vi "Flush Group Buffer.vi"(0 "TDMS File Ref in":refnum<k34>, 5 "Group Name":string, 7 "Channels":string[](array[string]), 9 "Group Buffer Data in":T1, 11 "error in (no error)":errorcluster) -> (4 "TDMS File Ref out":refnum<k34>, 8 "Flushed Data Size":u32, 10 "Group Buffer Data out":T1, 15 "error out":errorcluster)   [LabVIEW 2027, in "Embedded Data Logger Engine.lvlib"]
uses:
  Embedded Data Logger Engine.lvlib
  Group Buffer Data.ctl
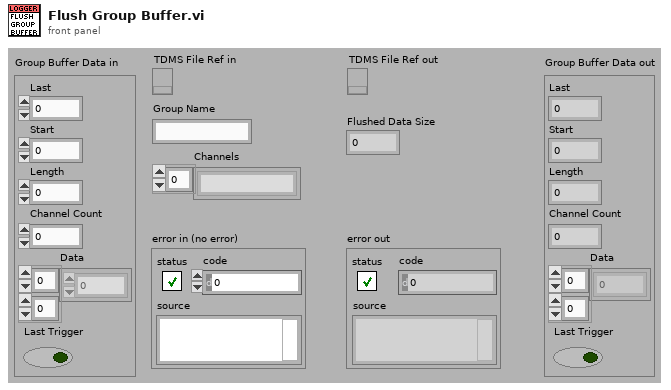
[diagram p1: front panel]
types:
  T1 = typedef "Embedded Data Logger Engine.lvlib/Group Buffer Data.ctl" = cluster{"Last":i32, "Start":i32, "Length":i32, "Channel Count":i32, "Data":dbl[][], "Last Trigger":bool}
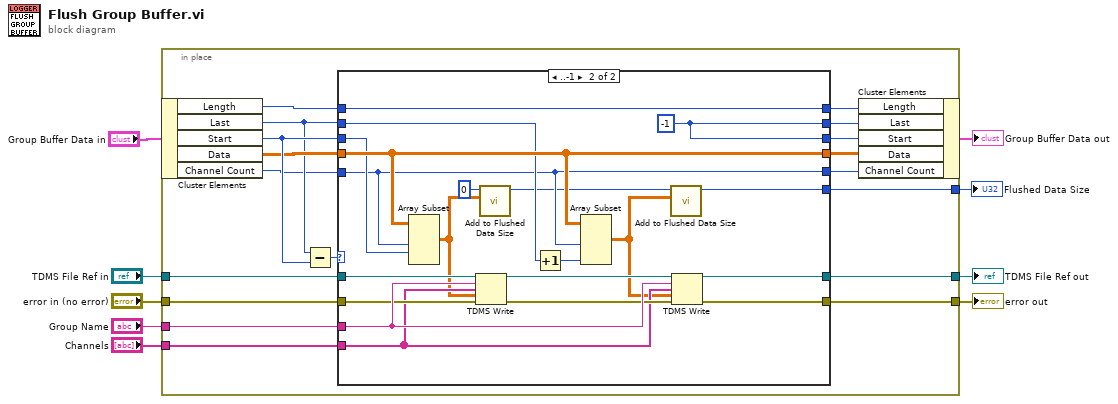
[diagram p0: block diagram]
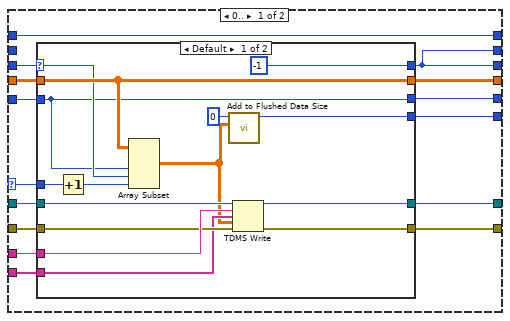
[diagram p2: hidden frame]
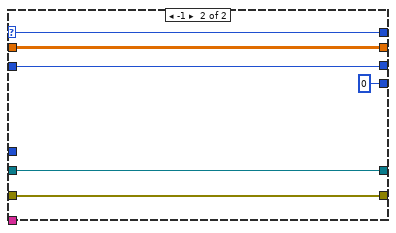
[diagram p3: hidden frame]
diagram:
  n1 = in-place {
    in-place-border: "error in (no error)" -> [w23]
    in-place-border: "TDMS File Ref in" -> [w26]
    in-place-border: [w25] -> w5
    in-place-border: [w24] -> w4
    in-place-border: "Group Name" -> [w22]
    in-place-border: "Channels" -> [w21]
    in-place-border: [w10] -> w1
    n2 = in-place-cluster #1("Group Buffer Data in") -> ("Length"=w14:i32, "Last"=w17:i32, "Start"=w27:i32, "Data"=w20:dbl[][], "Channel Count"=w11:i32)
    n3 = Subtract(x=w17, y=w27) -> (x-y=w18:i32)
    n4 = case shown="..-1" w18 {
      selector: w18 -> [w36 _]
      tunnel: w17 -> [_ w73]
      tunnel: [w38 w80] -> w16
      tunnel: [w38 w80] -> w15
      tunnel: w26 -> [w40 w81]
      tunnel: [w39 w77] -> w25
      tunnel: [w42 w76] -> w24
      tunnel: w23 -> [w41 w82]
      tunnel: w22 -> [w34 w83]
      tunnel: w21 -> [w33 w69]
      tunnel: w20 -> [w37 w75]
      tunnel: [w29 w75] -> w19
      tunnel: w27 -> [w32 w72]
      tunnel: w14 -> [w35 w74]
      tunnel: [w35 w74] -> w13
      tunnel: [w31 w70] -> w12
      tunnel: w11 -> [w30 w70]
      tunnel: [w28 w65] -> w10
      frame 0.. {
        n5 = case shown="Default" w32 {
          selector: w32 -> [w48 w63]
          tunnel: [w56 w61] -> w42
          tunnel: w41 -> [w55 w61]
          tunnel: w40 -> [w54 w62]
          tunnel: [w53 w62] -> w39
          tunnel: [-1 ("Start") w63] -> w38
          tunnel: w37 -> [w50 w59]
          tunnel: w36 -> [w51 _]
          tunnel: w34 -> [w57 _]
          tunnel: w33 -> [w46 _]
          tunnel: [w47 w60] -> w31
          tunnel: w30 -> [w47 w60]
          tunnel: [w50 w59] -> w29
          tunnel: [w44 u32 0 ("Flushed Data Size Out")] -> w28
          frame Default {
            n6 = Increment(x=w51) -> (x+1=w49:i32)
            n7 = Array Subset(array=w50, length (row)=w47, index (col)=w48, length (col)=w49) -> (w45:dbl[][])  [unwired: 1 in]
            n8 = call "Add to Flushed Data Size.vi"("TDMS Data Written"=w45, "Flushed Data Size In"=u32 0) -> ("Flushed Data Size Out"=w44:u32)  [unwired: 9 in]
            n9 = TDMS Write(0:w54, 5:w57, 7:w46, 9:w45, 11:w55) -> (4:w53:refnum<k34>, 15:w56:errorcluster)  [unwired: 1 in, 2 out]
          }
          frame -1 {
          }
        }
      }
      frame ..-1 {
        w80 = -1 ("Start")
        n10 = Array Subset(array=w75, length (row)=w70, index (col)=w72) -> (w68:dbl[][])  [unwired: 2 in]
        n11 = TDMS Write(0:w81, 5:w83, 7:w69, 9:w68, 11:w82) -> (4:w79:refnum<k34>, 15:w78:errorcluster)  [unwired: 1 in, 2 out]
        n12 = call "Add to Flushed Data Size.vi"("TDMS Data Written"=w68, "Flushed Data Size In"=u32 0) -> ("Flushed Data Size Out"=w67:u32)  [unwired: 9 in]
        n13 = Increment(x=w73) -> (x+1=w71:i32)
        n14 = Array Subset(array=w75, length (row)=w70, length (col)=w71) -> (w66:dbl[][])  [unwired: 2 in]
        n15 = call "Add to Flushed Data Size.vi"("TDMS Data Written"=w66, "Flushed Data Size In"=w67) -> ("Flushed Data Size Out"=w65:u32)  [unwired: 9 in]
        n16 = TDMS Write(0:w79, 5:w83, 7:w69, 9:w66, 11:w78) -> (4:w77:refnum<k34>, 15:w76:errorcluster)  [unwired: 1 in, 2 out]
      }
    }
    n17 = in-place-cluster #1("Length"=w13, "Last"=w16, "Start"=w15, "Data"=w19, "Channel Count"=w12) -> (→"Group Buffer Data out":T1)
  }
  "TDMS File Ref out" <- w5
  "error out" <- w4
  "Flushed Data Size" <- w1
